vi "Read Output Directory.vi"(8 "error in (no error)":errorcluster, 11 "SA Path in":refnum<class "SA 18GHz Path.lvclass">) -> (0 "error out":errorcluster, 2 "Output Directory":path, 3 "SA Path out":refnum<class "SA 18GHz Path.lvclass">)   [LabVIEW 2023, in "RFFixtureCharact.RFPM.lvlib" / "SA 18GHz Path.lvclass"]
uses:
  SA 18GHz Path.lvclass
  SA 18GHz Path.lvclass/SA 18GHz Path.ctl
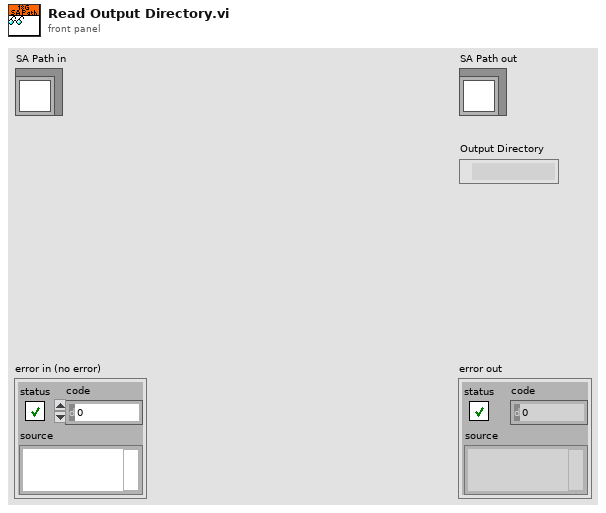
[diagram p1: front panel]
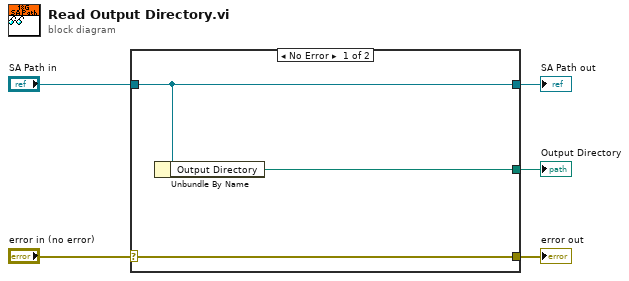
[diagram p0: block diagram]
diagram:
  n1 = case shown="No Error" "error in (no error)" {
    selector: "error in (no error)" -> [w8 w9]
    tunnel: [w8 w9] -> w4
    tunnel: [w7 w10] -> w2
    tunnel: "SA Path in" -> [w7 w10]
    tunnel: [w6 _] -> w1
    frame No Error {
      n2 = Unbundle By Name(w7) -> ("Output Directory"=w6:path)
    }
    frame Error {
    }
  }
  "error out" <- w4
  "SA Path out" <- w2
  "Output Directory" <- w1
